vi "uiControlsMgr.vi"(8 "error in (no error)":errorcluster, 9 "Captions File":string, 11 "VI reference":refnum<vi>) -> (0 "error out":errorcluster, 3 "uiControlsMgr out":refnum<class "uiControlsMgr.lvclass">)   [LabVIEW 2020, in "UI Controls Manager.lvlib" / "uiControlsMgr.lvclass"]
uses:
  uiControlsMgr.lvclass
  uiControlsMgr.lvclass/uiControlsMgr.ctl
  <vilib>/Utility/file.llb/Read Delimited Spreadsheet (string).vi
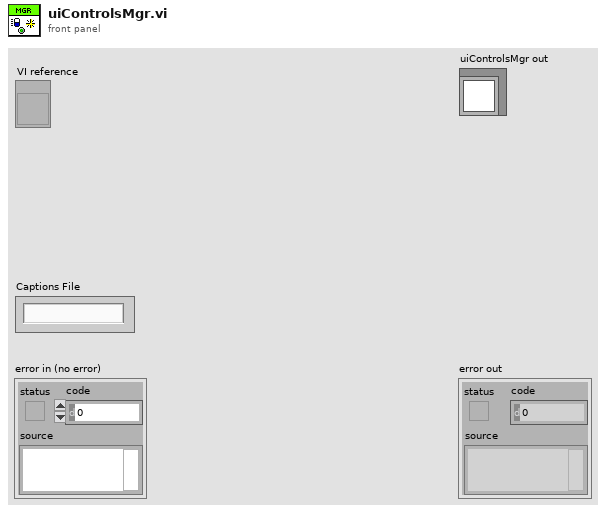
[diagram p1: front panel]
types:
  T1 = cluster{"Caption":string, "Ctl Refnum":refnum<vi>}
  T2 = map{string, cluster{"Caption":string, "Ctl Refnum":refnum<vi>}}
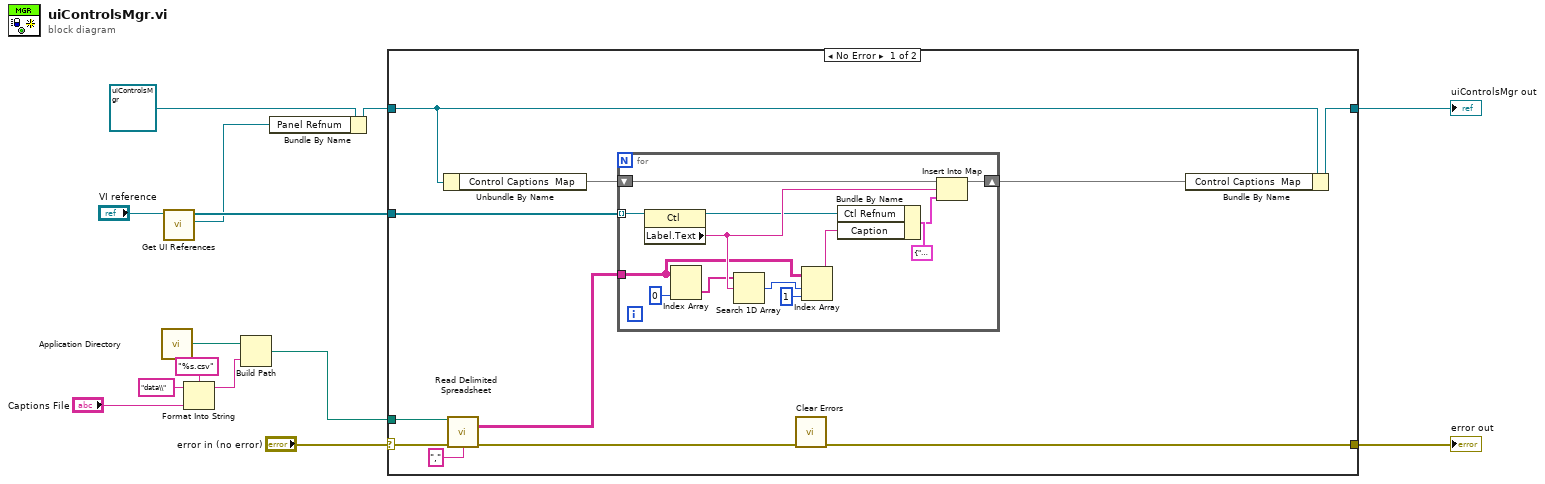
[diagram p0: block diagram]
diagram:
  n1 = call <vilib>:"Application Directory.vi"() -> ("Application Directory"=w10:path)
  n2 = call "Get UI References.vi"("VI reference"="VI reference") -> ("reference out"=w1:refnum<vi>, "Controls[]"=w4:refnum<vi>[])  [unwired: 8 in, 1 out]
  n3 = Format Into String(format string="%s.csv", initial string="data\\", "Captions File") -> (resulting string=w6:string)  [unwired: 1 in, 1 out]
  n4 = Build Path(base path=w10, name or relative path=w6) -> (appended path=w5:path)
  n5 = Bundle By Name(cluster=refnum<class "uiControlsMgr.lvclass"> refnum ("uiControlsMgr in"), "Panel Refnum"=w1) -> (w2:refnum<class "uiControlsMgr.lvclass">)
  n6 = case shown="No Error" "error in (no error)" {
    selector: "error in (no error)" -> [w25 w40]
    tunnel: [w15 w40] -> w13
    tunnel: [w22 w39] -> w11
    tunnel: w2 -> [w24 w39]
    tunnel: w4 -> [w16 _]
    tunnel: w5 -> [w19 _]
    frame No Error {
      n7 = Unbundle By Name(w24) -> ("Control Captions  Map"=w23:T2)
      n8 = call-poly <vilib>:"Read Delimited Spreadsheet.vi"("file path (dialog if empty)"=w19, "error in (no error)"=w25, "delimiter (\\t)"="," ("delimiter (\\t)")) -> ("all rows"=w17:string[][], "error out"=w20:errorcluster)  [unwired: 7 in, 4 out]
      n9 = for {
        tunnel: w16 -> [w36] mode=indexing
        shift-right: [w37] -> w21
        shift-left: w23 -> [w38]
        tunnel: w17 -> [w31]
        n10 = property class="Ctl"(reference=w36) -> (reference out=w27:refnum<vi>, "Label.Text"=w35:string)  [unwired: 1 in, 1 out]
        n11 = Index Array(array=w31, index (col)=0 ("disabled index (col)")) -> (element=w33:string[])  [unwired: 1 in]
        n12 = Search 1D Array(1D array=w33, element=w35) -> (index of element=w30:i32)  [unwired: 1 in]
        n13 = Index Array(array=w31, index (row)=w30, index (col)=1 ("disabled index (col)")) -> (element=w26:string)
        n14 = Bundle By Name(cluster=T1 {"Caption"="", "Ctl Refnum"=refnum} ("Control Data"), "Ctl Refnum"=w27, "Caption"=w26) -> (w28:T1)
        n15 = Insert Into Map(map in=w38, key=w35, value=w28) -> (map out=w37:T2)  [unwired: 2 out]
      }
      n16 = call <vilib>:"Clear Errors.vi"("error in (no error)"=w20) -> ("error out"=w15:errorcluster)  [unwired: 5 in, 1 out]
      n17 = Bundle By Name(cluster=w24, "Control Captions  Map"=w21) -> (w22:refnum<class "uiControlsMgr.lvclass">)
    }
    frame Error {
    }
  }
  "error out" <- w13
  "uiControlsMgr out" <- w11
